vi "Calibration-Splash-Normalizing.vi"(8 "error in (no error)":errorcluster) -> (0 "error out":errorcluster)   [LabVIEW 2013, in "Calibration-RunTest.lvclass"]
uses:
  Calibration-RunTest.lvclass
panel:
  in  "x":dbl=70.0 format="%#_13g"
  out "Normalizing Data":u8(slide) scale=0.0..20.0
  # "Please Wait While the data is Normalized"
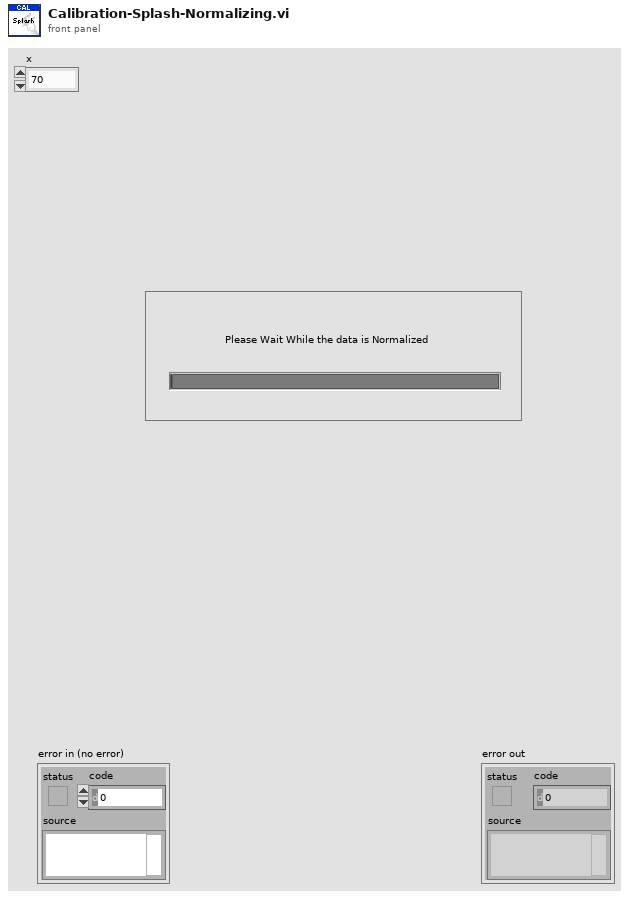
[diagram p1: front panel]
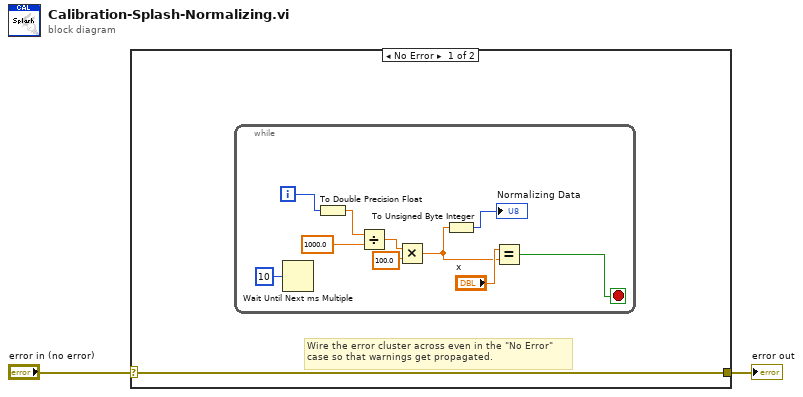
[diagram p0: block diagram]
diagram:
  n1 = case shown="No Error" "error in (no error)" {
    selector: "error in (no error)" -> [w3 w14]
    tunnel: [w3 w14] -> w1
    frame No Error {
      # "Wire the error cluster across even in the \"No Error\"\ncase so that warnings get propagated."
      n2 = while {
        i -> [w12]
        stop <- w4 stop-if-true
        n3 = Wait Until Next ms Multiple(millisecond multiple=u32 10) -> ()  [unwired: 1 out]
        n4 = To Double Precision Float(number=w12) -> (double precision float=w11:dbl)
        n5 = Divide(x=w11, y=1000.0) -> (x/y=w9:dbl)
        n6 = Multiply(x=w9, y=100.0) -> (x*y=w5:dbl)
        n7 = To Unsigned Byte Integer(number=w5) -> (unsigned 8bit integer=→"Normalizing Data":u8)
        n8 = Equal?(x="x", y=w5) -> (x = y?=w4:bool)
      }
    }
    frame Error {
    }
  }
  "error out" <- w1
